vi "Export time-lapse snippet.vi"(11 "AVI File Path":path) -> ()   [LabVIEW 2013]
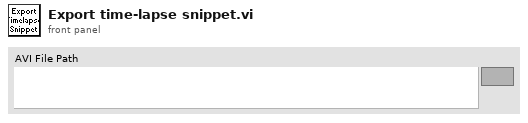
[diagram p1: front panel]
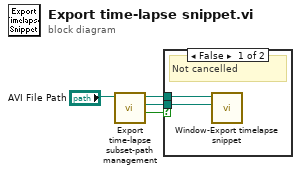
[diagram p0: block diagram]
diagram:
  n1 = call "Export time-lapse subset-path management.vi"("AVI path in"="AVI File Path") -> ("cancelled"=w3:bool, "New folder path"=w1:path, "Existing AVI path"=w2:path)  [unwired: 8 in]
  n2 = case shown="False" w3 {
    tunnel: w2 -> [w6 _]
    tunnel: w1 -> [w5 _]
    frame False {
      # "Not cancelled"
      n3 = call "Window-Export timelapse snippet.vi"("New folder path"=w5, "Existing AVI path"=w6) -> ()  [unwired: 10 in]
    }
    frame True {
      # "Cancelled"
    }
  }
